vi "Turn Crank.vi"(0 "reference in":refnum<class "Sold Out State.lvclass">, 5 "error in (no error)":errorcluster) -> (14 "reference out":refnum<class "Sold Out State.lvclass">, 19 "error out":errorcluster)   [LabVIEW 2013, in "Sold Out State.lvclass"]
uses:
  Sold Out State.lvclass
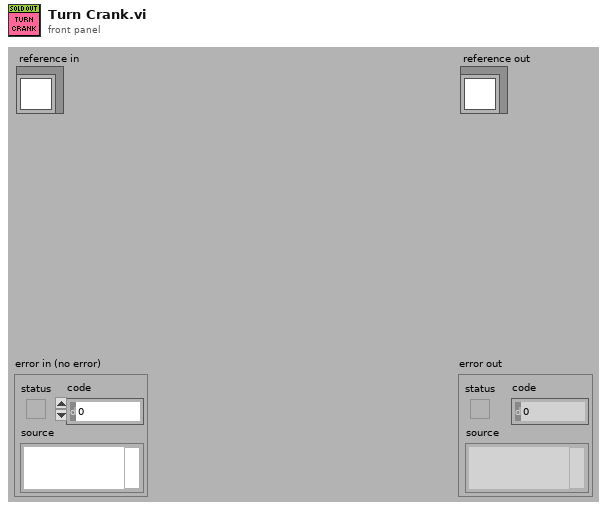
[diagram p1: front panel]
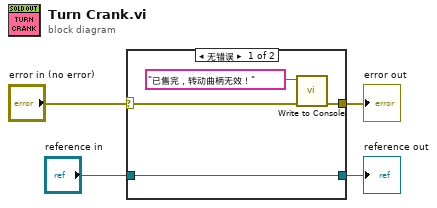
[diagram p0: block diagram]
diagram:
  n1 = case shown="无错误" "error in (no error)" {
    selector: "error in (no error)" -> [w7 w10]
    tunnel: [w6 w10] -> w3
    tunnel: [w8 w9] -> w1
    tunnel: "reference in" -> [w8 w9]
    frame No Error {
      n2 = call "Write to Console.vi"("error in (no error)"=w7, "Input"="已售完，转动曲柄无效！") -> ("error out"=w6:errorcluster)  [unwired: 9 in]
    }
    frame Error {
    }
  }
  "error out" <- w3
  "reference out" <- w1
